vi "Activate.vi"(8 "error in (no error)":errorcluster, 11 "Abstract License in":refnum<class "Software License Manager.lvclass">) -> (0 "error out":errorcluster, 1 "ok?":bool, 3 "Abstract License out":refnum<class "Software License Manager.lvclass">)   [LabVIEW 2021, in "Software License Manager.lvclass"]
uses:
  Software License Manager.lvclass
  Software License Manager.lvclass/Software License Manager.ctl
  Board/Board.lvclass/Board.ctl
  Board/Read Product ID.vi
  Board/Read Host Name.vi
  <vilib>/httpClient/POSTBuffer.vi
  <vilib>/httpClient/LabVIEWHTTPClient.lvlib
  Board/Board.lvclass
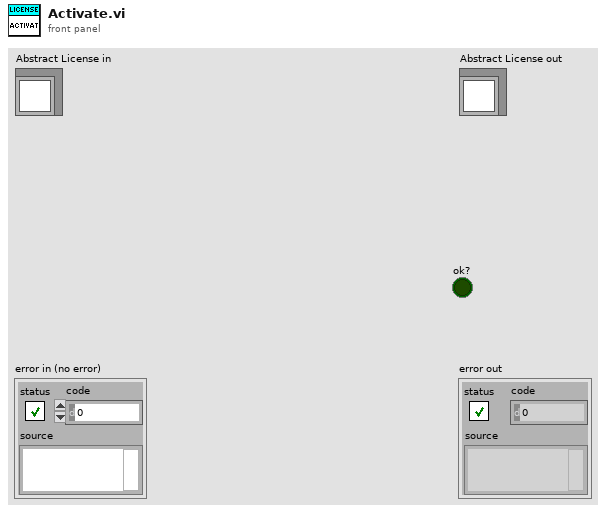
[diagram p1: front panel]
types:
  T1 = typedef "LabVIEWHTTPClient.lvlib/ClientHandle.ctl" = refnum<k1>
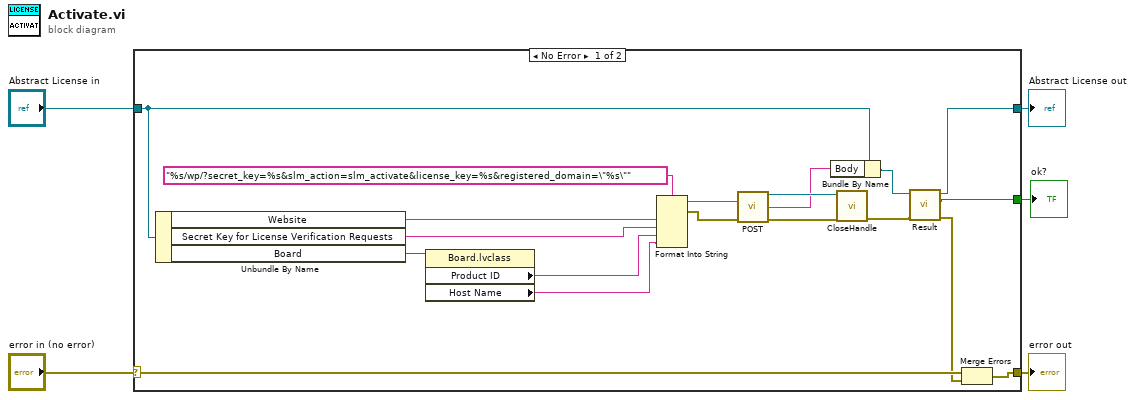
[diagram p0: block diagram]
diagram:
  n1 = case shown="No Error" "error in (no error)" {
    selector: "error in (no error)" -> [w10 w26]
    tunnel: [w16 w26] -> w4
    tunnel: [w7 w25] -> w2
    tunnel: "Abstract License in" -> [w15 w25]
    tunnel: [w8 _] -> w1
    frame No Error {
      n2 = Unbundle By Name(w15) -> ("Website"=w23:string, "Secret Key for License Verification Requests"=w6:string, "Board"=w22:refnum<class "Board.lvclass">)
      n3 = property class="Board.lvclass"(reference=w22) -> ("Product ID"=w21:string, "Host Name"=w20:string)  [unwired: 1 in, 2 out]
      n4 = Format Into String(format string="%s/wp/?secret_key=%s&slm_action=slm_activate&license_key=%s&registered_domain=\"%s\"", w23, w6, w21, w20) -> (resulting string=w13:string, error out=w17:errorcluster)  [unwired: 2 in]
      n5 = call-poly <vilib>:"POST.vi"("url"=w13, "error in (no error)"=w17) -> ("client handle out"=w19:T1, "body"=w14:string, "error out"=w18:errorcluster)  [unwired: 10 in, 1 out]
      n6 = Bundle By Name(cluster=w15, "Body"=w14) -> (w12:refnum<class "Software License Manager.lvclass">)
      n7 = call <vilib>:"CloseHandle.vi"("client handle"=w19, "error in (no error)"=w18) -> ("error out"=w11:errorcluster)  [unwired: 13 in]
      n8 = call-dynamic "Result.vi"("error in (no error)"=w11, "Software License Manager in"=w12) -> ("error out"=w9:errorcluster, "ok?"=w8:bool, "Software License Manager out"=w7:refnum<class "Software License Manager.lvclass">)  [unwired: 6 in, 1 out]
      n9 = Merge Errors(w10, w9) -> (w16:errorcluster)
    }
    frame Error {
    }
  }
  "error out" <- w4
  "Abstract License out" <- w2
  "ok?" <- w1
